vi "SENS_CORR_RVEL_COAX.vi"(0 "VISA IN":refnum<visa-resource-name>, 1 "Velocity Factor":dbl, 5 "error in":errorcluster, 7 "Channel":i32) -> (14 "VISA Out":refnum<visa-resource-name>, 19 "error out":errorcluster)   [LabVIEW 2018, in "PNA-X.lvlib"]
doc: "SENSe<cnum>:CORRection:RVELocity:COAX <num> \n1638\n\n(Read-Write) Sets the velocity factor to be used with Electrical Delay and Port Extensions. \nParameters \n<cnum> Any existing channel number. If unspecified, value is set to 1 \n<num> Velocity factor. Choose a number between 0 and 10 \n(.66 polyethylene dielectric; .7 teflon dielectric) \nExamples SENS:CORR:RVEL:COAX .66 \nsense2:correction:rvelocity:coax .70 \nQuery Syntax SENSe<cnum>:CORRection:RVELocity:COAX? \nReturn Type Numeric \nDefault 1 \nSENSe:CORRection:SFORward[:STATe] <boolean> \n(Read-Write) Sets the direction a calibration will be performed when only one set of standards is used. \nUse SENSe:CORRection:TSTandards[:STATe] OFF to specify that only one set of standards will be \nused. \nParameters \n<boolean> ON (1) - FORWARD direction of a 2-port calibration will be performed \nOFF (0) - REVERSE direction of a 2-port calibration will be performed \nExamples SENS:CORR:SFOR 1 \nsense:correction:sforward:state 0 \nSee an example using this command \nQuery Syntax SENSe:CORRection:SFORward[:STATe]? \nReturn Type Boolean \nDefault ON"
uses:
  PNA-X.lvlib
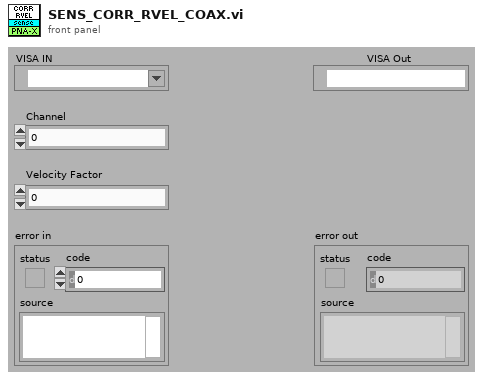
[diagram p1: front panel]
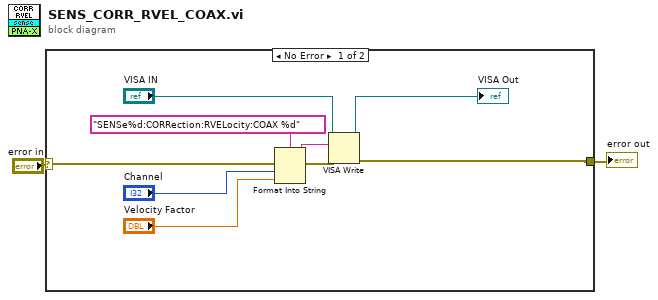
[diagram p0: block diagram]
diagram:
  n1 = case shown="No Error" "error in" {
    selector: "error in" -> [w11 w12]
    tunnel: [w6 w12] -> w1
    frame No Error {
      n2 = Format Into String(format string="SENSe%d:CORRection:RVELocity:COAX %d" ("Cmdline"), error in=w11, "Channel", "Velocity Factor") -> (resulting string=w9:string, error out=w10:errorcluster)  [unwired: 1 in]
      n3 = VISA Write(VISA resource name="VISA IN", write buffer=w9, error in (no error)=w10) -> (VISA resource name out=→"VISA Out":refnum<visa-resource-name>, error out=w6:errorcluster)  [unwired: 1 out]
    }
    frame Error {
    }
  }
  "error out" <- w1
